vi "Choose location.vi"(9 "Map dimensions":dbl[](array[numeric]), 10 "robot location":dbl[](array[numeric]), 11 "Dispaly map":u16[][](array[ring])) -> (3 "target location":dbl[](array[numeric]))   [LabVIEW 2015]
panel:
  out "Boolean 8":bool
  out "Boolean 7":bool
  out "Boolean 6":bool
  out "Boolean 5":bool
  out "Boolean 4":bool
  out "Boolean 3":bool
  out "Boolean 2":bool
  out "Boolean":bool
  out "x":dbl
  out "Priority map":dbl[][](array[numeric])
  out "distances":dbl[](array[numeric])
  out "Highest priority locations":i32[][](array[numeric])
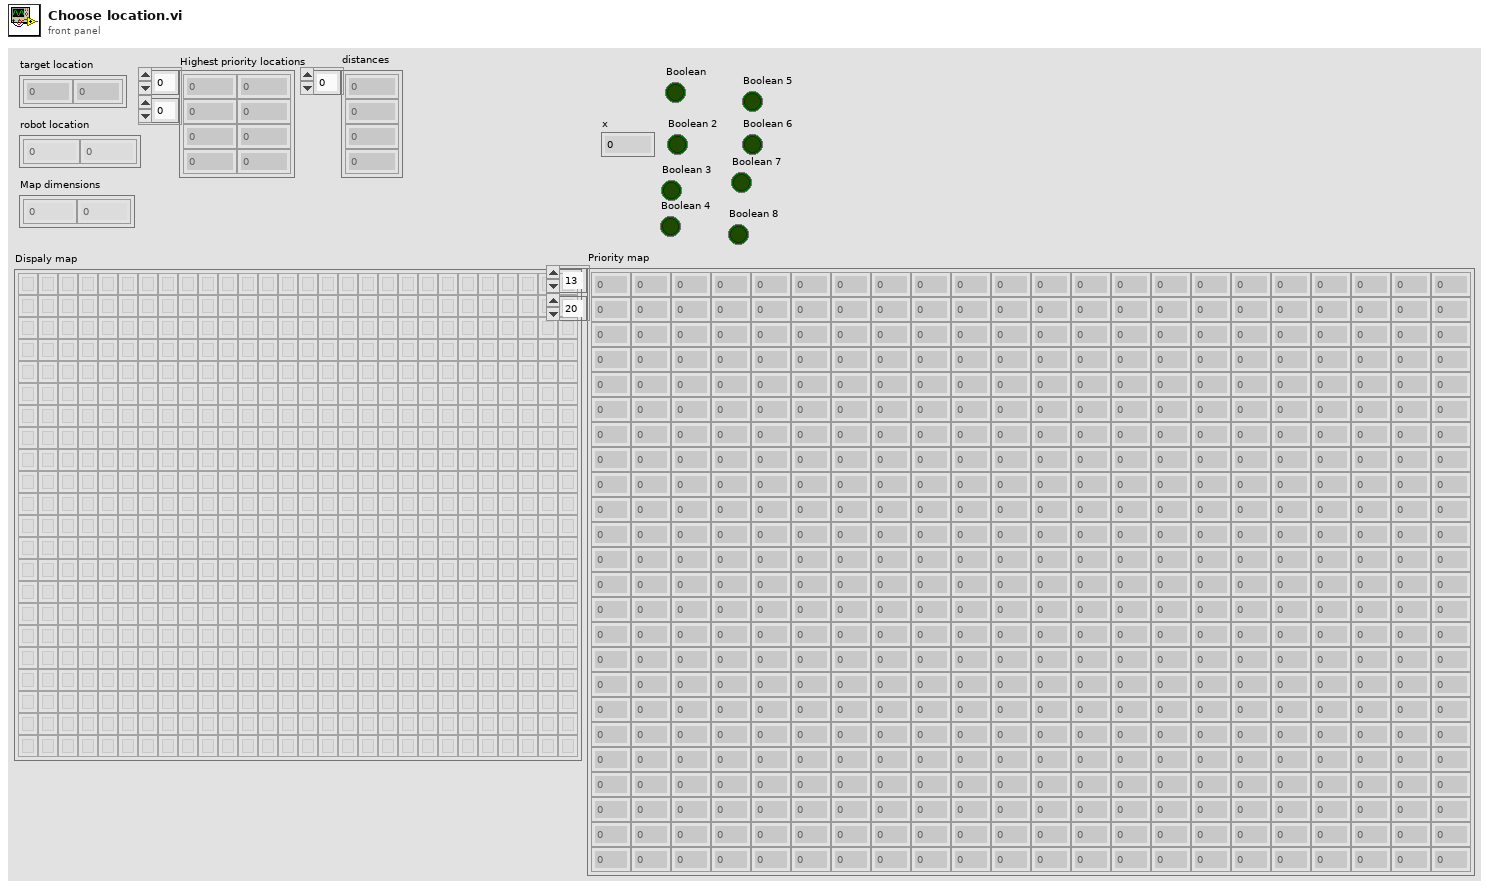
[diagram p1: front panel]
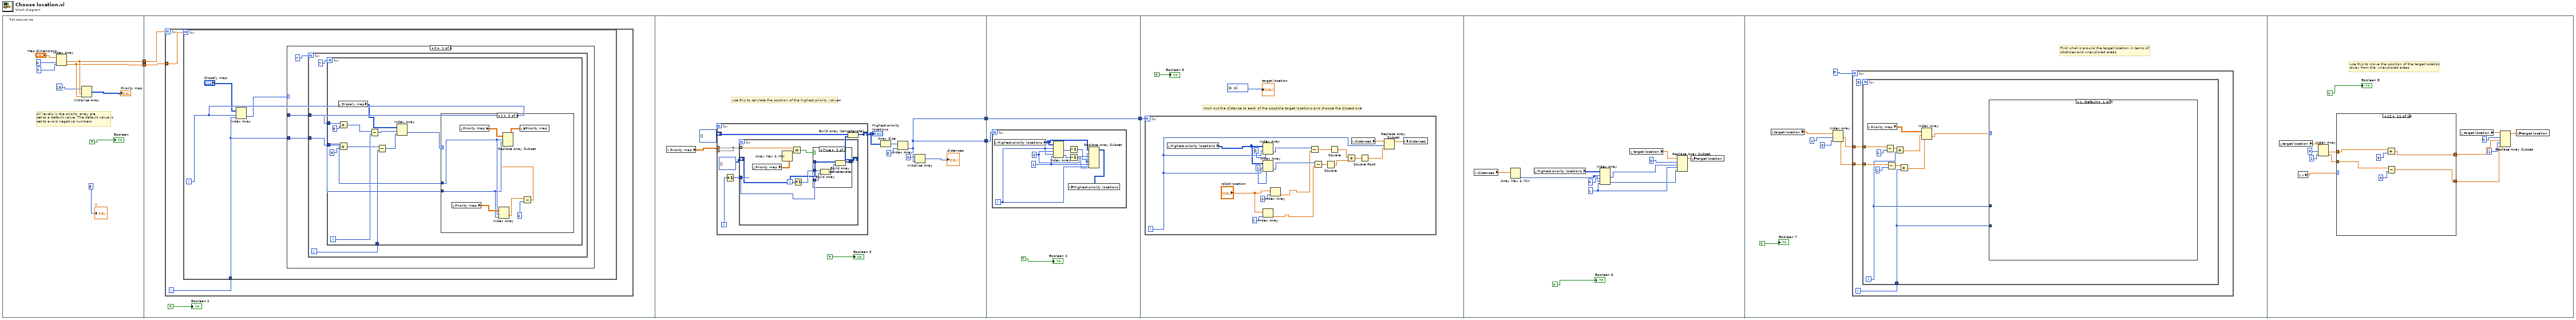
[diagram p0: block diagram]
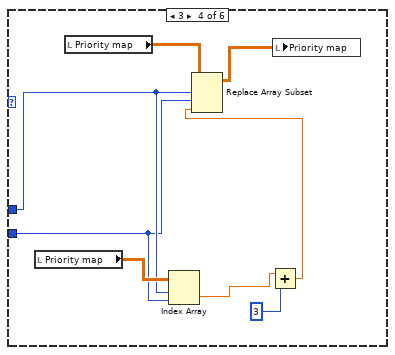
[diagram p4: hidden frame]
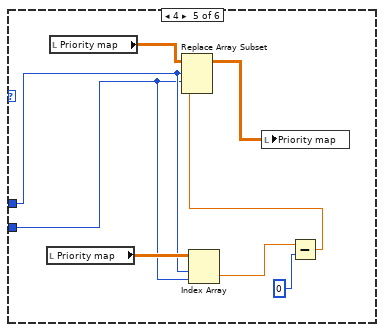
[diagram p5: hidden frame]
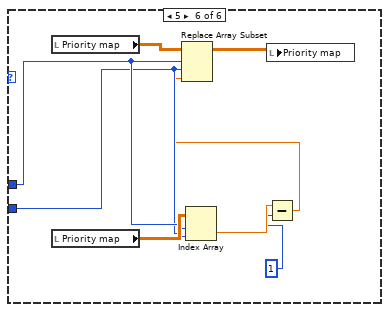
[diagram p6: hidden frame]
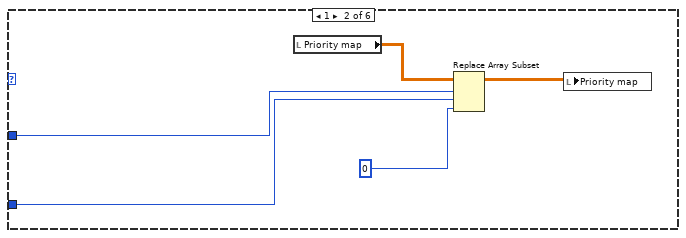
[diagram p7: hidden frame]
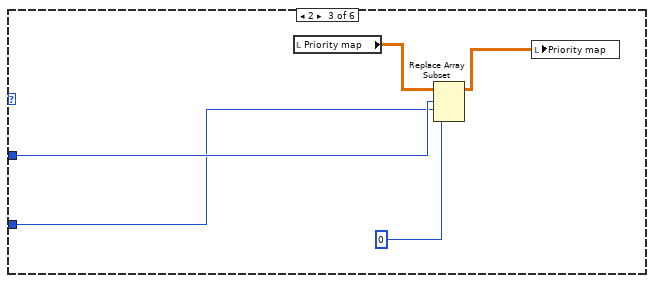
[diagram p8: hidden frame]
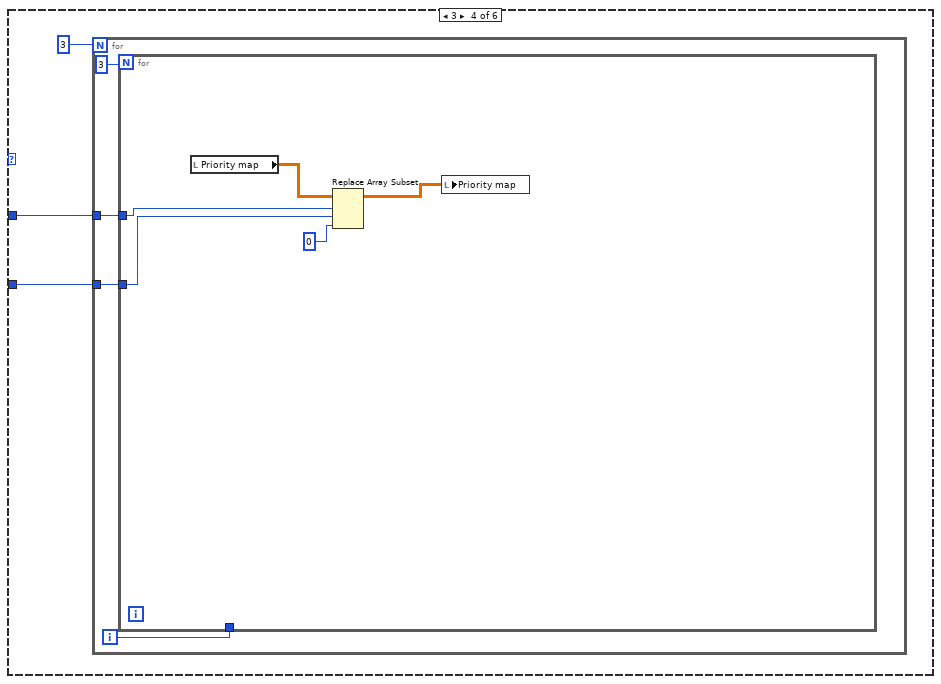
[diagram p9: hidden frame]
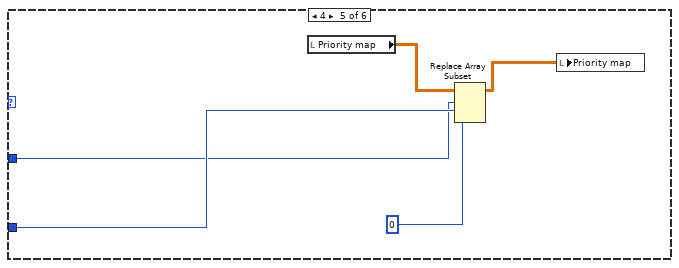
[diagram p10: hidden frame]
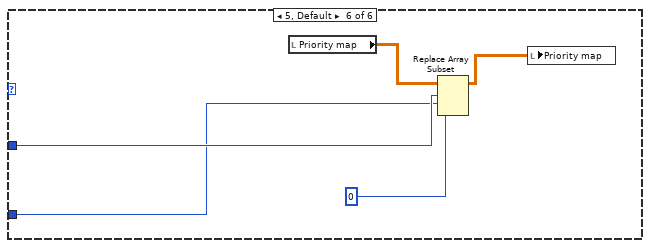
[diagram p11: hidden frame]
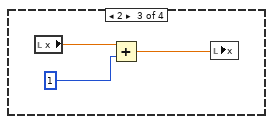
[diagram p16: hidden frame]
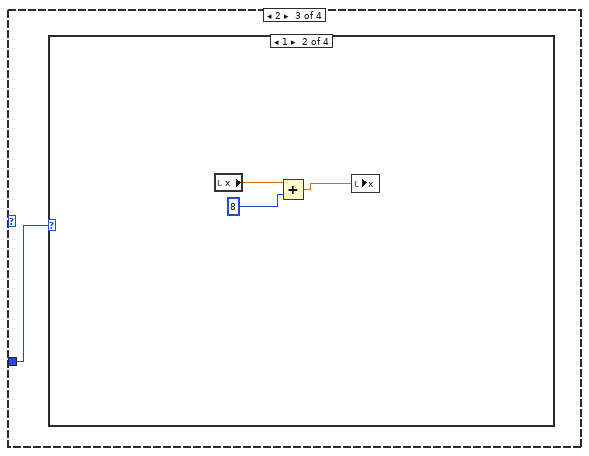
[diagram p18: hidden frame]
diagram:
  n1 = flat-sequence {
    tunnel: [w11] -> w5
    tunnel: [w10] -> w4
    tunnel: w5 -> [w17]
    tunnel: w4 -> [w16]
    tunnel: [w108] -> w3
    tunnel: [w108] -> w1
    tunnel: w3 -> [w140]
    tunnel: [w140] -> w2
    tunnel: w1 -> [w139]
    tunnel: w2 -> [w151]
    frame #0 {
      # "All levels in the priority array are \nset to a default value. The default value is \nset to avoid negative numbers"
      n2 = Index Array(array="Map dimensions", index #1=0, index #2=1) -> (element #1=w11:dbl, element #2=w10:dbl)
      n3 = Initialize Array(15, w11, w10) -> (→"Priority map":i32[][])
      "x" <- 5
      "Boolean" <- TRUE
    }
    frame #1 {
      n4 = for {
        N: w17 -> [_]
        tunnel: w16 -> [w18]
        i -> [w19]
        n5 = for {
          N: w18 -> [_]
          tunnel: w19 -> [w23]
          i -> [w22]
          n6 = Index Array(array="Dispaly map", index (row)=w22, index (col)=w23) -> (element=w21:u16)
          n7 = case shown="0" w21 {
            tunnel: w23 -> [w26 w76 w82 w87 w99 w103]
            tunnel: w22 -> [w25 w75 w83 w86 w98 w104]
            frame 0 {
              n8 = for {
                N: 7 -> [_]
                tunnel: w26 -> [w30]
                tunnel: w25 -> [w29]
                i -> [w27]
                n9 = for {
                  N: 7 -> [_]
                  tunnel: w30 -> [w39]
                  tunnel: w29 -> [w38]
                  tunnel: w27 -> [w34]
                  i -> [w36]
                  n10 = local read "Dispaly map"() -> (w42:u16[][])
                  n11 = Add(x=w38, y=5) -> (x+y=w37:i32)
                  n12 = Add(x=w39, y=5) -> (x+y=w35:i32)
                  n13 = Subtract(x=w37, y=w36) -> (x-y=w32:i32)
                  n14 = Subtract(x=w35, y=w34) -> (x-y=w33:i32)
                  n15 = Index Array(array=w42, index (row)=w32, index (col)=w33) -> (element=w31:u16)
                  n16 = case shown="1" w31 {
                    tunnel: w39 -> [_ w46 _ w55 w62 w70]
                    tunnel: w38 -> [_ w47 _ w56 w63 w71]
                    frame 0, Default {
                    }
                    frame 1 {
                      n17 = local read "Priority map"() -> (w50:dbl[][])
                      n18 = local read "Priority map"() -> (w49:dbl[][])
                      n19 = Index Array(array=w50, index (row)=w47, index (col)=w46) -> (element=w45:dbl)
                      n20 = Subtract(x=w45, y=2) -> (x-y=w43:dbl)
                      n21 = Replace Array Subset(array=w49, new element=w43, index (row)=w47, index (col)=w46) -> (w48:dbl[][])
                      n22 = local write "Priority map"(w48) -> ()
                    }
                    frame 2 {
                    }
                    frame 3 {
                      n23 = local read "Priority map"() -> (w57:dbl[][])
                      n24 = local read "Priority map"() -> (w58:dbl[][])
                      n25 = Index Array(array=w57, index (row)=w56, index (col)=w55) -> (element=w54:dbl)
                      n26 = Add(x=w54, y=3) -> (x+y=w52:dbl)
                      n27 = Replace Array Subset(array=w58, new element=w52, index (row)=w56, index (col)=w55) -> (w53:dbl[][])
                      n28 = local write "Priority map"(w53) -> ()
                    }
                    frame 4 {
                      n29 = local read "Priority map"() -> (w64:dbl[][])
                      n30 = local read "Priority map"() -> (w66:dbl[][])
                      n31 = Index Array(array=w64, index (row)=w63, index (col)=w62) -> (element=w61:dbl)
                      n32 = Subtract(x=w61, y=0) -> (x-y=w60:dbl)
                      n33 = Replace Array Subset(array=w66, new element=w60, index (row)=w63, index (col)=w62) -> (w65:dbl[][])
                      n34 = local write "Priority map"(w65) -> ()
                    }
                    frame 5 {
                      n35 = local read "Priority map"() -> (w72:dbl[][])
                      n36 = local read "Priority map"() -> (w74:dbl[][])
                      n37 = Index Array(array=w74, index (row)=w71, index (col)=w70) -> (element=w69:dbl)
                      n38 = Subtract(x=w69, y=1) -> (x-y=w68:dbl)
                      n39 = Replace Array Subset(array=w72, new element=w68, index (row)=w71, index (col)=w70) -> (w73:dbl[][])
                      n40 = local write "Priority map"(w73) -> ()
                    }
                  }
                }
              }
            }
            frame 1 {
              n41 = local read "Priority map"() -> (w79:dbl[][])
              n42 = Replace Array Subset(array=w79, new element=0, index (row)=w75, index (col)=w76) -> (w78:dbl[][])
              n43 = local write "Priority map"(w78) -> ()
            }
            frame 2 {
              n44 = local read "Priority map"() -> (w84:dbl[][])
              n45 = Replace Array Subset(array=w84, new element=0, index (row)=w83, index (col)=w82) -> (w81:dbl[][])
              n46 = local write "Priority map"(w81) -> ()
            }
            frame 3 {
              n47 = for {
                N: 3 -> [_]
                tunnel: w87 -> [w91]
                tunnel: w86 -> [w90]
                i -> [w88]
                n48 = for {
                  N: 3 -> [_]
                  tunnel: w91 -> [w92]
                  tunnel: w90 -> [w93]
                  tunnel: w88 -> [_]
                  n49 = local read "Priority map"() -> (w96:dbl[][])
                  n50 = Replace Array Subset(array=w96, new element=0, index (row)=w93, index (col)=w92) -> (w95:dbl[][])
                  n51 = local write "Priority map"(w95) -> ()
                }
              }
            }
            frame 4 {
              n52 = local read "Priority map"() -> (w101:dbl[][])
              n53 = Replace Array Subset(array=w101, new element=0, index (row)=w98, index (col)=w99) -> (w100:dbl[][])
              n54 = local write "Priority map"(w100) -> ()
            }
            frame 5, Default {
              n55 = local read "Priority map"() -> (w106:dbl[][])
              n56 = Replace Array Subset(array=w106, new element=0, index (row)=w104, index (col)=w103) -> (w105:dbl[][])
              n57 = local write "Priority map"(w105) -> ()
            }
          }
        }
      }
      "Boolean 2" <- TRUE
    }
    frame #2 {
      # "use this to calulate the position of the highest priority values"
      n58 = local read "Priority map"() -> (w114:dbl[][])
      n59 = for {
        tunnel: w114 -> [w117] mode=indexing
        shift-right: [w120] -> w111
        shift-left: i32[][] [] -> [w118]
        tunnel: [w117] -> _ mode=indexing
        i -> [w122]
        n60 = Increment(x=w122) -> (x+1=w121:i32)
        n61 = for {
          tunnel: w117 -> [w131] mode=indexing
          tunnel: w121 -> [w127]
          shift-right: [w126] -> w119
          shift-left: i32[][] [] -> [w125]
          i -> [w129]
          n62 = local read "Priority map"() -> (w123:dbl[][])
          n63 = Array Max & Min(array=w123) -> (max value=w124:dbl)  [unwired: 3 out]
          n64 = Equal?(x=w131, y=w124) -> (x = y?=w130:bool)
          n65 = Increment(x=w129) -> (x+1=w128:i32)
          n66 = case shown="True" w130 {
            tunnel: w128 -> [_ w137]
            tunnel: w127 -> [_ w136]
            tunnel: [w132 w134] -> w126
            tunnel: w125 -> [w132 w133]
            frame False {
            }
            frame True {
              n67 = Build Array(w137, w136) -> (w135:i32[])
              n68 = Build Array (concatenate)(w133, w135) -> (w134:i32[][])
            }
          }
        }
        n69 = Build Array (concatenate)(w118, w119) -> (w120:i32[][])
      }
      "Highest priority locations" <- w111
      n70 = Array Size(array=w111) -> (size(s)=w110:i32[])
      n71 = Index Array(array=w110, index=0) -> (element=w108:i32)
      n72 = Initialize Array(0, w108) -> (→"distances":i32[])
      "Boolean 3" <- TRUE
    }
    frame #3 {
      n73 = for {
        N: w139 -> [_]
        i -> [w143]
        w145 = 1
        w144 = 0
        n74 = local read "Highest priority locations"() -> (w147:i32[][])
        n75 = Index Array(array=w147, index (row) #1=w143, index (col) #1=w144, index (row) #2=w143, index (col) #2=w145) -> (element #1=w149:i32, element #2=w148:i32)
        n76 = Decrement(x=w149) -> (x-1=w142:i32)
        n77 = Decrement(x=w148) -> (x-1=w141:i32)
        n78 = Replace Array Subset(array=w147, new element #1=w142, index (row) #1=w143, index (col) #1=w144, new element #2=w141, index (row) #2=w143, index (col) #2=w145) -> (w146:i32[][])
        n79 = local write "Highest priority locations"(w146) -> ()
      }
      "Boolean 4" <- TRUE
    }
    frame #4 {
      # "Work out the distance to each of the possible target locations and choose the closest one"
      n80 = for {
        N: w151 -> [_]
        i -> [w159]
        n81 = local read "Highest priority locations"() -> (w157:i32[][])
        n82 = Index Array(array=w157, index (row)=w159, index (col)=0) -> (element=w169:i32)
        n83 = Index Array(array=w157, index (row)=w159, index (col)=1) -> (element=w168:i32)
        n84 = Index Array(array="robot location", index=1) -> (element=w153:dbl)
        n85 = Index Array(array="robot location", index=0) -> (element=w154:dbl)
        n86 = Subtract(x=w169, y=w154) -> (x-y=w167:dbl)
        n87 = Subtract(x=w168, y=w153) -> (x-y=w162:dbl)
        n88 = Square(x=w162) -> (x^2=w166:dbl)
        n89 = Square(x=w167) -> (x^2=w165:dbl)
        n90 = Add(x=w165, y=w166) -> (x+y=w164:dbl)
        n91 = local read "distances"() -> (w155:dbl[])
        n92 = Square Root(x=w164) -> (sqrt(x)=w163:dbl)
        n93 = Replace Array Subset(array=w155, new element=w163, index=w159) -> (w156:dbl[])
        n94 = local write "distances"(w156) -> ()
      }
      "target location" <- i32[] [0, 0]
      "Boolean 5" <- TRUE
    }
    frame #5 {
      w175 = 1
      n95 = local read "distances"() -> (w182:dbl[])
      n96 = Array Max & Min(array=w182) -> (min index (indices)=w176:i32)  [unwired: 3 out]
      n97 = local read "Highest priority locations"() -> (w177:i32[][])
      n98 = Index Array(array=w177, index (row) #1=w176, index (col) #1=0, index (row) #2=w176, index (col) #2=w175) -> (element #1=w174:i32, element #2=w173:i32)
      n99 = local read "target location"() -> (w180:dbl[])
      n100 = Replace Array Subset(array=w180, new element #1=w174, index #1=0, new element #2=w173, index #2=w175) -> (w181:dbl[])
      n101 = local write "target location"(w181) -> ()
      "Boolean 6" <- TRUE
    }
    frame #6 {
      # "Find what is around the target location in terms of \nobsticles and unexplored areas"
      n102 = local read "target location"() -> (w189:dbl[])
      n103 = Index Array(array=w189, index #1=1, index #2=0) -> (element #1=w185:dbl, element #2=w184:dbl)
      n104 = for {
        N: 3 -> [_]
        tunnel: w185 -> [w192]
        tunnel: w184 -> [w191]
        i -> [w190]
        n105 = for {
          N: 3 -> [_]
          tunnel: w192 -> [w202]
          tunnel: w191 -> [w201]
          tunnel: w190 -> [w195]
          i -> [w196]
          n106 = local read "Priority map"() -> (w205:dbl[][])
          n107 = Subtract(x=w202, y=1) -> (x-y=w200:dbl)
          n108 = Subtract(x=w201, y=1) -> (x-y=w199:dbl)
          n109 = Add(x=w200, y=w196) -> (x+y=w198:dbl)
          n110 = Add(x=w199, y=w195) -> (x+y=w197:dbl)
          n111 = Index Array(array=w205, index (row)=w198, index (col)=w197) -> (element=w194:dbl)
          n112 = case shown="1, Default" w194 {
            tunnel: w196 -> [_ w207]
            tunnel: w195 -> [_ w206]
            frame 1, Default {
            }
            frame 0 {
              n113 = case shown="1" w207 {
                tunnel: w206 -> [_ w208 w212 w219]
                frame 0, Default {
                }
                frame 1 {
                  n114 = case shown="1" w208 {
                    frame 0, Default {
                    }
                    frame 1 {
                    }
                    frame 2 {
                      n115 = local read "x"() -> (w211:dbl)
                      n116 = Add(x=w211, y=1) -> (x+y=w210:dbl)
                      n117 = local write "x"(w210) -> ()
                    }
                    frame 3 {
                    }
                  }
                }
                frame 2 {
                  n118 = case shown="1" w212 {
                    frame 0, Default {
                    }
                    frame 1 {
                      n119 = local read "x"() -> (w215:dbl)
                      n120 = Add(x=w215, y=8) -> (x+y=w214:dbl)
                      n121 = local write "x"(w214) -> ()
                    }
                    frame 2 {
                    }
                    frame 3 {
                      n122 = local read "x"() -> (w218:dbl)
                      n123 = Add(x=w218, y=2) -> (x+y=w217:dbl)
                      n124 = local write "x"(w217) -> ()
                    }
                  }
                }
                frame 3 {
                  n125 = case shown="1" w219 {
                    frame 0, Default {
                    }
                    frame 1 {
                    }
                    frame 2 {
                      n126 = local read "x"() -> (w222:dbl)
                      n127 = Add(x=w222, y=4) -> (x+y=w221:dbl)
                      n128 = local write "x"(w221) -> ()
                    }
                    frame 3 {
                    }
                  }
                }
              }
            }
          }
        }
      }
      "Boolean 7" <- TRUE
    }
    frame #7 {
      # "use this to move the position of the target location\naway from the  unexplored areas"
      n129 = local read "target location"() -> (w232:dbl[])
      n130 = local read "x"() -> (w235:dbl)
      n131 = Index Array(array=w232, index #1=0, index #2=1) -> (element #1=w225:dbl, element #2=w224:dbl)
      n132 = case shown="12" w235 {
        tunnel: [w236 w240 w244 w249 w255 w260 w263 w268 w271 w277 w283 w289 w290 w296 w304 w309] -> w227
        tunnel: [w237 w239 w245 w250 w256 w261 w262 w269 w272 w276 w284 w288 w291 w298 w305 w310] -> w226
        tunnel: w225 -> [w237 w238 w246 w251 w257 w261 w265 w269 w273 w279 w285 w288 w295 w299 w306 w311]
        tunnel: w224 -> [w236 w241 w244 w248 w254 w260 w264 w268 w270 w278 w282 w289 w294 w297 w303 w308]
        frame 0, Default {
        }
        frame 1 {
          n133 = Add(x=w238, y=0) -> (x+y=w239:dbl)
          n134 = Add(x=w241, y=3) -> (x+y=w240:dbl)
        }
        frame 2 {
          n135 = Subtract(x=w246, y=3) -> (x-y=w245:dbl)
        }
        frame 3 {
          n136 = Subtract(x=w251, y=3) -> (x-y=w250:dbl)
          n137 = Add(x=w248, y=3) -> (x+y=w249:dbl)
        }
        frame 4 {
          n138 = Add(x=w257, y=0) -> (x+y=w256:dbl)
          n139 = Subtract(x=w254, y=3) -> (x-y=w255:dbl)
        }
        frame 5 {
        }
        frame 6 {
          n140 = Subtract(x=w265, y=3) -> (x-y=w262:dbl)
          n141 = Subtract(x=w264, y=3) -> (x-y=w263:dbl)
        }
        frame 7 {
        }
        frame 8 {
          n142 = Add(x=w273, y=3) -> (x+y=w272:dbl)
          n143 = Add(x=w270, y=0) -> (x+y=w271:dbl)
        }
        frame 9 {
          n144 = Add(x=w279, y=3) -> (x+y=w276:dbl)
          n145 = Add(x=w278, y=3) -> (x+y=w277:dbl)
        }
        frame 12 {
          n146 = Add(x=w285, y=3) -> (x+y=w284:dbl)
          n147 = Subtract(x=w282, y=3) -> (x-y=w283:dbl)
        }
        frame 14 {
        }
        frame 20 {
          n148 = Add(x=w295, y=3) -> (x+y=w291:dbl)
          n149 = Add(x=w294, y=3) -> (x+y=w290:dbl)
        }
        frame 30 {
          n150 = Subtract(x=w299, y=3) -> (x-y=w298:dbl)
          n151 = Add(x=w297, y=3) -> (x+y=w296:dbl)
        }
        frame 40 {
          n152 = Add(x=w306, y=3) -> (x+y=w305:dbl)
          n153 = Subtract(x=w303, y=3) -> (x-y=w304:dbl)
        }
        frame 50 {
          n154 = Subtract(x=w311, y=3) -> (x-y=w310:dbl)
          n155 = Subtract(x=w308, y=3) -> (x-y=w309:dbl)
        }
      }
      n156 = local read "target location"() -> (w234:dbl[])
      n157 = Replace Array Subset(array=w234, new element #1=w226, index #1=0, new element #2=w227, index #2=1) -> (w233:dbl[])
      n158 = local write "target location"(w233) -> ()
      "Boolean 8" <- TRUE
    }
  }
